vi "MapCoordstoXY.vi"(1 "Coordinates":cluster{"Raw X":dbl, "Raw Y":dbl}, 3 "XYGraph Refnum":refnum<vi>) -> (8 "Y(graph)":dbl, 9 "X (graph)":dbl)   [LabVIEW 2010]
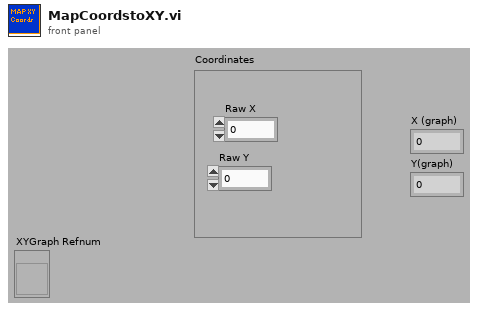
[diagram p1: front panel]
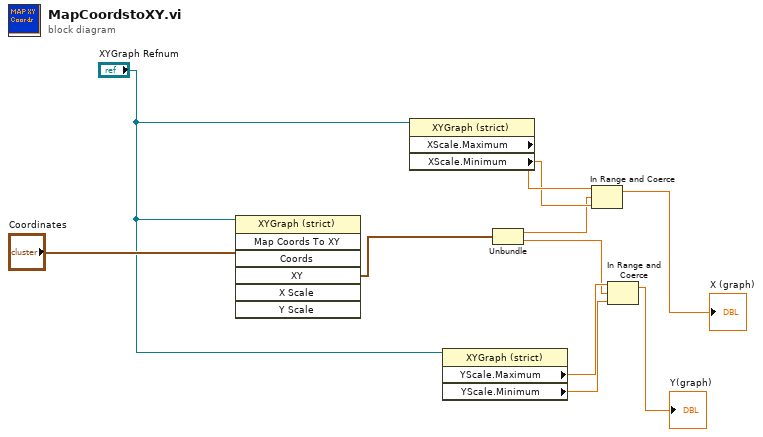
[diagram p0: block diagram]
diagram:
  n1 = invoke on="Invoke Node" class="XYGraph (strict)" method="Map Coords To XY"(reference="XYGraph Refnum", "Coords"="Coordinates") -> ("XY"=w2:cluster{"X":dbl, "Y":dbl})  [unwired: 5 in, 6 out]
  n2 = property on="Property Node" class="XYGraph (strict)"(reference="XYGraph Refnum") -> ("XScale.Maximum"=w10:dbl, "XScale.Minimum"=w9:dbl)  [unwired: 1 in, 2 out]
  n3 = property on="Property Node" class="XYGraph (strict)"(reference="XYGraph Refnum") -> ("YScale.Maximum"=w7:dbl, "YScale.Minimum"=w6:dbl)  [unwired: 1 in, 2 out]
  n4 = Unbundle(w2) -> ("X"=w8:dbl, "Y"=w5:dbl)
  n5 = In Range and Coerce(upper limit=w10, x=w8, lower limit=w9) -> (coerced(x)=→"X (graph)":dbl)  [unwired: 1 out]
  n6 = In Range and Coerce(upper limit=w7, x=w5, lower limit=w6) -> (coerced(x)=→"Y(graph)":dbl)  [unwired: 1 out]
